vi "Process Signals with a Filter Bank Tree.vi"() -> ()   [LabVIEW 2023]
doc: "This example demonstrates how to decompose and reconstruct signals with a filter bank tree.\n\nComplete the following steps to use this example.\n1) Specify an <b>Input Signal</b>.\n2) Run this VI.\n3) Observe the <b>Signals</b> graph. The output signal is a delayed version of the input signal. \n4) Observe the <b>Reconstruction Error</b> graph. The magnitude of the reconstruction error is small."
uses:
  <vilib>/addons/Digital Filter Design/Process.llb/DFD Integer Delay (Array).vi
  <vilib>/addons/Digital Filter Design/NI_DigFilter_FilterBank.lvlib
  <vilib>/addons/Digital Filter Design/NI_DigFilterLicensed.lvlib
  <vilib>/Analysis/NI_AALBase.lvlib
panel:
  out "Reconstruction Error":dbl[](graph)
  in  "Input Signal":enum16{"White Noise", "Sine", "Chirp"}(ring)=enum."Sine"
  out "Signals":dbl[][](graph)
  # "Select Help»Show Context Help and move the cursor over the VI icon for more information."
  # "Select Help>>Show Context Help and move the cursor over the VI icon for more information."
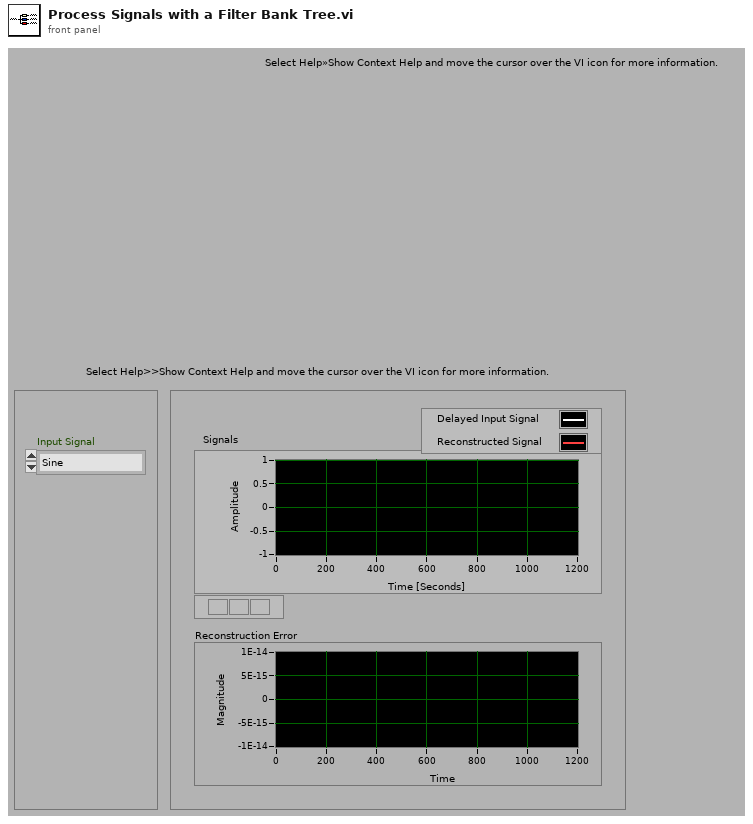
[diagram p1: front panel]
types:
  T1 = typedef "NI_DigFilter_FilterBank.lvlib/DFD Filter Bank Obj.ctl" = cluster{"mFBank_AnalysisFilters":T2[], "mFBank_SynthesisFilters":T2[], "mFBank_#Bands":i32, "mFBank_ProcMethod":T7, "mFBank_Coeffs":dbl[], "mFBank_Gain":dbl, "mFBank_Delay":i32, "mFBank_Type":T8}
  T2 = typedef "NI_DigFilterLicensed.lvlib/DFD Multirate Filter Obj.ctl" = cluster{"mMRate_Structure":enum16{"CIC", "FIR", "IIR", "Lattice"}, "mMRate_Mode":T3, "mMRate_Factor":i32, "mMRate_FIRParams":cluster{"mMRate_FIR_H":dbl[], "mMRate_FIR_IsNyquist?":bool, "mMRate_FIR_IsSymmetric?":bool}, "mMRate_CICParams":cluster{"mMRate_CIC_#Stage":i32, "mMRate_CIC_Lag":i32, "mMRate_CIC_Type":enum16{"Lowpass", "Highpass"}}, "mMRate_Order":i32, "mMRate_Version":string, "mMRate_Comments":string, "mMRate_RationalFactor":cluster{"mMRate_L":i32, "mMRate_M":i32}, "mMRate_Fs":dbl, "mMRate_Quantized?":bool, "mMRate_QFilterGain":dbl, "mMRate_CoefWl":i16, "mMRate_Scaling":cluster{"mMRate_ScaleByPowerOf2?":bool, "mMRate_ScaleType":T4}, "mMRate_InputWl":i16, "mMRate_OutputWl":i16, "mMRate_OutputMode":T5, "mMRate_MultMode":T6, "mMRate_BitPruning":bool, "mMRate_GainWl":i16, "mMRate_OutputFwl":i16, "mMRate_SumIwl":i16, "mMRate_InputIwl ":i16, "mMRate_SumWl":i16, "mMRate_CoefIwl":i16}
  T3 = typedef "NI_DigFilterLicensed.lvlib/DFD Multirate Mode.ctl" = i16
  T4 = typedef "NI_DigFilterLicensed.lvlib/DFD Coef Norm Type.ctl" = enum16{"No Norm", "Time Domain 1-Norm", "Time Domain 2-Norm", "Time Domain Inf-Norm"}
  T5 = typedef "NI_DigFilterLicensed.lvlib/DFD Round-off Mode.ctl" = enum16{"Nearest", "Truncation"}
  T6 = typedef "NI_DigFilterLicensed.lvlib/DFD FXP MRate Multiply Mode.ctl" = enum16{"Truncated", "Full"}
  T7 = typedef "NI_DigFilter_FilterBank.lvlib/DFD Filter Bank Processing Method.ctl" = enum16{"General", "2-Band QMF Lattice", "Cosine-Modulated"}
  T8 = typedef "NI_DigFilter_FilterBank.lvlib/DFD Filter Bank Type.ctl" = u16
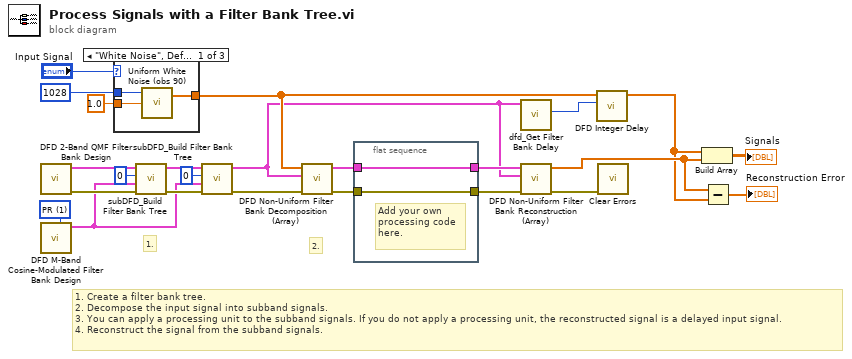
[diagram p0: block diagram]
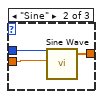
[diagram p2: hidden frame]
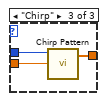
[diagram p3: hidden frame]
diagram:
  w17 = u16 1 items=["NPR", "PR"] ("PR?")
  # "2."
  # "1."
  # "1. Create a filter bank tree.\n2. Decompose the input signal into subband signals.\n3. You can apply a processing unit to the subband signals. If you do not apply a processing unit, the reconstructed signal is a delayed input signal.\n4. Reconstruct the signal from the subband signals."
  n1 = call <vilib>:"DFD 2-Band QMF Filter Bank Design.vi"() -> ("error out"=w24:errorcluster, "filter bank out"=w15:T1)  [unwired: 9 in, 1 out]
  n2 = call <vilib>:"DFD M-Band Cosine-Modulated Filter Bank Design.vi"("signal reconstruction"=w17) -> ("filter bank out"=w16:T1)  [unwired: 9 in, 1 out]
  n3 = case shown="\"White Noise\", Default" "Input Signal" {
    tunnel: [w27 w30 w33] -> w5
    tunnel: 1028 ("samples") -> [w26 w29 w32]
    tunnel: 1.0 -> [w25 w28 w31]
    frame "White Noise", Default {
      n4 = call <vilib>:"Uniform White Noise (obs 90).vi"("amplitude"=w25, "samples"=w26) -> ("uniform white noise"=w27:dbl[])  [unwired: 1 in, 1 out]
    }
    frame "Sine" {
      n5 = call <vilib>:"Sine Wave.vi"("samples"=w29, "amplitude"=w28) -> ("sine wave"=w30:dbl[])  [unwired: 3 in, 2 out]
    }
    frame "Chirp" {
      n6 = call <vilib>:"Chirp Pattern.vi"("amplitude"=w31, "samples"=w32) -> ("Chirp Pattern"=w33:dbl[])  [unwired: 2 in, 1 out]
    }
  }
  n7 = call "subDFD_Build Filter Bank Tree.vi"("error in (no error)"=w24, "bank to append"=w16, "branch index"=0, "tree in"=w15) -> ("error out"=w23:errorcluster, "tree out"=w19:T1)  [unwired: 6 in]
  n8 = call "subDFD_Build Filter Bank Tree.vi"("error in (no error)"=w23, "bank to append"=w16, "branch index"=0, "tree in"=w19) -> ("error out"=w10:errorcluster, "tree out"=w2:T1)  [unwired: 6 in]
  n9 = call "DFD Non-Uniform Filter Bank Decomposition (Array).vi"("error in (no error)"=w10, "filter bank in"=w2, "x"=w5) -> ("error out"=w14:errorcluster, "M bands"=w12:cluster{"band":dbl[]}[])  [unwired: 7 in]
  n10 = flat-sequence {
    tunnel: w14 -> [w35]
    tunnel: [w35] -> w13
    tunnel: w12 -> [w34]
    tunnel: [w34] -> w11
    frame #0 {
      # "Add your own \nprocessing code\nhere."
    }
  }
  n11 = call <vilib>:"dfd_Get Filter Bank Delay.vi"("bank in"=w2) -> ("delay"=w1:i32)  [unwired: 8 in, 2 out]
  n12 = call "DFD Non-Uniform Filter Bank Reconstruction (Array).vi"("error in (no error)"=w13, "filter bank in"=w2, "M bands"=w11) -> ("error out"=w4:errorcluster, "y"=w18:dbl[])  [unwired: 7 in]
  n13 = call-poly <vilib>:"DFD Integer Delay.vi"("delay"=w1, "signal in"=w5) -> ("signal out"=w3:dbl[])  [unwired: 8 in, 1 out]
  n14 = call <vilib>:"Clear Errors.vi"("error in (no error)"=w4) -> ()  [unwired: 5 in, 2 out]
  n15 = Build Array(w3, w18) -> (→"Signals":dbl[][])
  n16 = Subtract(x=w18, y=w3) -> (x-y=→"Reconstruction Error":dbl[])
